vi "LEP_RV_LaunchFarmLogin.vi"(0 "error in (no error)":errorcluster, 1 "uV Licensed":bool=TRUE, 2 "build on exit":bool) -> (7 "error out":errorcluster, 9 "Connect to a network compile server":bool, 10 "OK":bool)   [LabVIEW 2011]
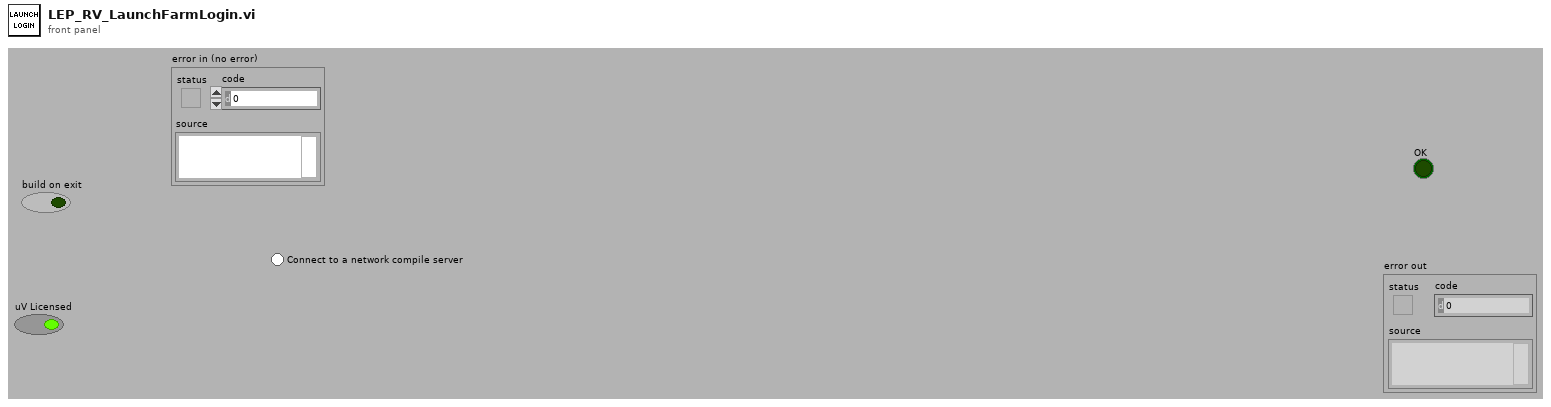
[diagram p1: front panel]
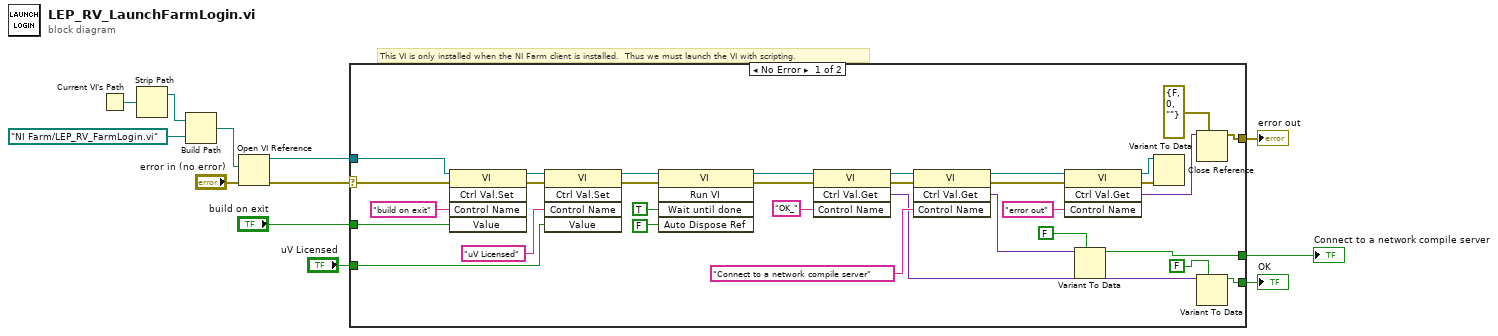
[diagram p0: block diagram]
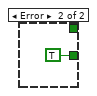
[diagram p2: hidden frame]
diagram:
  # "This VI is only installed when the NI Farm client is installed.  Thus we must launch the VI with scripting."
  n1 = Current VI's Path() -> (path=w11:path)
  n2 = Strip Path(path=w11) -> (stripped path=w10:path)  [unwired: 1 out]
  n3 = Build Path(base path=w10, name or relative path=path "NI Farm/LEP_RV_FarmLogin.vi") -> (appended path=w9:path)
  n4 = Open VI Reference(vi path=w9, error in (no error)="error in (no error)") -> (vi reference=w8:refnum<vi>, error out=w7:errorcluster)  [unwired: 4 in]
  n5 = case shown="No Error" w7 {
    selector: w7 -> [w21 _]
    tunnel: w8 -> [w20 _]
    tunnel: [w32 _] -> w3
    tunnel: [w31 TRUE ("OK")] -> w1
    tunnel: [w30 _] -> w2
    tunnel: "build on exit" -> [w22 _]
    tunnel: "uV Licensed" -> [w23 _]
    frame No Error {
      n6 = invoke class="VI" method="Ctrl Val.Set"(reference=w20, error in=w21, "Control Name"="build on exit", "Value"=w22) -> (reference out=w28:refnum<vi>, error out=w29:errorcluster)  [unwired: 1 in, 3 out]
      n7 = invoke class="VI" method="Ctrl Val.Set"(reference=w28, error in=w29, "Control Name"="uV Licensed", "Value"=w23) -> (reference out=w26:refnum<vi>, error out=w27:errorcluster)  [unwired: 1 in, 3 out]
      n8 = invoke class="VI" method="Run VI"(reference=w26, error in=w27, "Wait until done"=TRUE ("Wait Until Done"), "Auto Dispose Ref"=FALSE ("Auto Dispose Reference")) -> (reference out=w42:refnum<vi>, error out=w41:errorcluster)  [unwired: 1 in, 3 out]
      n9 = invoke class="VI" method="Ctrl Val.Get"(reference=w42, error in=w41, "Control Name"="OK_") -> (reference out=w38:refnum<vi>, error out=w37:errorcluster, "Get Control Value Variant"=w17:variant)  [unwired: 1 in, 1 out]
      n10 = invoke class="VI" method="Ctrl Val.Get"(reference=w38, error in=w37, "Control Name"="Connect to a network compile server") -> (reference out=w40:refnum<vi>, error out=w39:errorcluster, "Get Control Value Variant"=w16:variant)  [unwired: 1 in, 1 out]
      n11 = invoke class="VI" method="Ctrl Val.Get"(reference=w40, error in=w39, "Control Name"="error out") -> (reference out=w19:refnum<vi>, error out=w18:errorcluster, "Get Control Value Variant"=w33:variant)  [unwired: 1 in, 1 out]
      n12 = Variant To Data(type=FALSE ("Connect to a network compile server"), Variant=w16) -> (data=w30:bool)  [unwired: 1 in, 1 out]
      n13 = Close Reference(reference=w19, error in (no error)=w18) -> ()  [unwired: 1 out]
      n14 = Variant To Data(type=errorcluster {"status"=FALSE, "code"=0, "source"=""} ("error out"), Variant=w33) -> (data=w32:errorcluster)  [unwired: 1 in, 1 out]
      n15 = Variant To Data(type=FALSE ("OK"), Variant=w17) -> (data=w31:bool)  [unwired: 1 in, 1 out]
    }
    frame Error {
    }
  }
  "OK" <- w1
  "error out" <- w3
  "Connect to a network compile server" <- w2
